vi "DAQ Write Safe Outputs.vi"(8 "error in (no error)":errorcluster) -> (0 "error out":errorcluster)   [LabVIEW 2022 SP3]
uses:
  <vilib>/DAQmx/write.llb/DAQmx Write (Analog 1D DBL NChan 1Samp).vi
  Globals/Global - Configuration Options.vi
  <vilib>/DAQmx/create/channels.llb/DAQmx Create Virtual Channel.vi
  <vilib>/DAQmx/miscellaneous.llb/DAQmx Fill In Error Info.vi
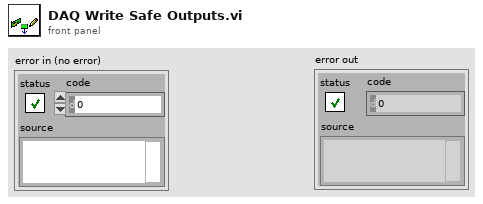
[diagram p1: front panel]
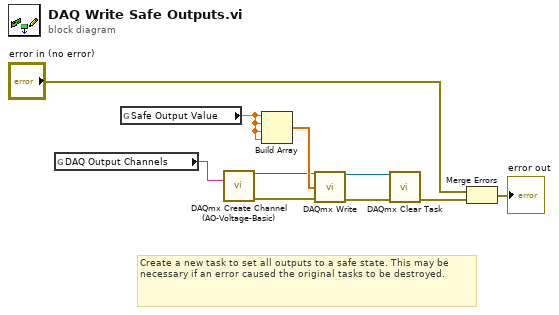
[diagram p0: block diagram]
diagram:
  # "Create a new task to set all outputs to a safe state. This may be necessary if an error caused the original tasks to be destroyed."
  n1 = global read "Global - Configuration Options.vi" "DAQ Output Channels"() -> (w1:tag)
  n2 = global read "Global - Configuration Options.vi" "Safe Output Value"() -> (w7:dbl)
  n3 = call-poly <vilib>:"DAQmx Create Channel (AO-Voltage-Basic).vi"("physical channels"=w1) -> ("task out"=w5:refnum<k21>, "error out"=w6:errorcluster)  [unwired: 13 in]
  n4 = Build Array(w7, w7, w7, w7) -> (w8:dbl[])
  n5 = call-poly <vilib>:"DAQmx Write.vi"("task/channels in"=w5, "data"=w8, "error in"=w6) -> ("task out"=w10:refnum<k21>, "error out"=w9:errorcluster)  [unwired: 10 in, 1 out]
  n6 = call <vilib>:"DAQmx Clear Task.vi"("task in"=w10, "error in"=w9) -> ("error out"=w4:errorcluster)  [unwired: 13 in]
  n7 = Merge Errors("error in (no error)", w4) -> (→"error out":errorcluster)
